vi "411x_Current _Chan Config Dialog.vi"(8 "error in (no error)":errorcluster, 10 "Item Ref out":T1=18446744073709551615 format="%.0x", 11 "Data Entry Limits:Maximum":dbl) -> (0 "error out":errorcluster, 1 "sense (out)":T2=1008 items=["Local"=1008, "Remote"=1009], 2 "Voltage Limit (out)":dbl, 3 "Initial Current Value (out)":dbl, 4 "Cancel (out)":bool, 5 "Number of Current Channels to Add? (out)":i16, 7 "Item Ref out":T1 format="%.0x")   [LabVIEW 2023, in "NI PXIe-411x PS Custom Device.lvlib"]
uses:
  NI PXIe-411x PS Custom Device.lvlib
  <instrlib>/niDCPower/nidcpower.llb/niDCPower Sense.ctl
  <vilib>/NI VeriStand/Custom Device API/Custom Device Item Ref.ctl
  411x_Global.vi
  <vilib>/NI VeriStand/Custom Device API/Get Item Property (Boolean).vi
  <vilib>/NI VeriStand/Custom Device API/Custom Device API.lvlib
panel:
  in  "Cancel":bool
  in  "OK Button":bool
  in  "Voltage Limit":dbl format="%.4f"
  in  "Initial Current Value":dbl
  in  "sense":T2=1008 caption="Sense" items=["Local"=1008, "Remote"=1009]
  in  "Number of Current Channels to Add?":i16
  # "Current Channels"
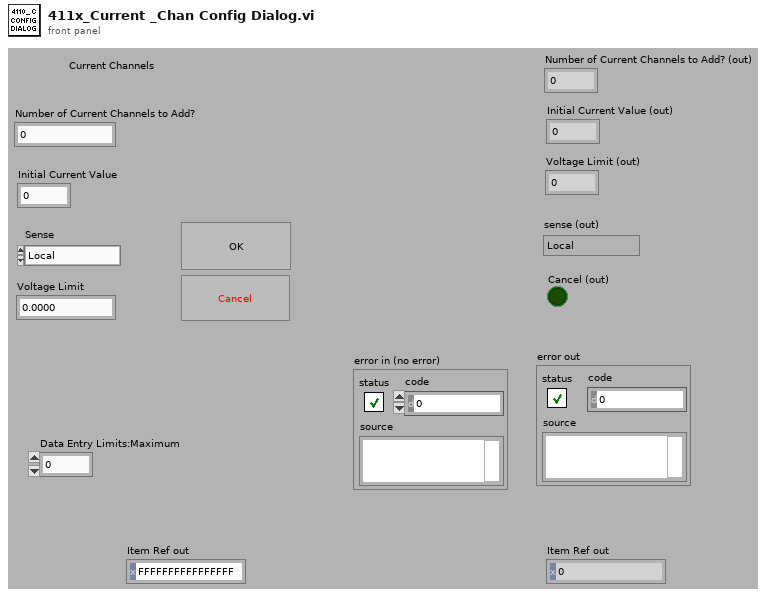
[diagram p1: front panel]
types:
  T1 = typedef "Custom Device API.lvlib/Custom Device Item Ref.ctl" = u64
  T2 = typedef "niDCPower Sense.ctl" = i32
  T3 = cluster{"V_min":dbl, "V_max":dbl, "I_min":dbl, "I_max":dbl}
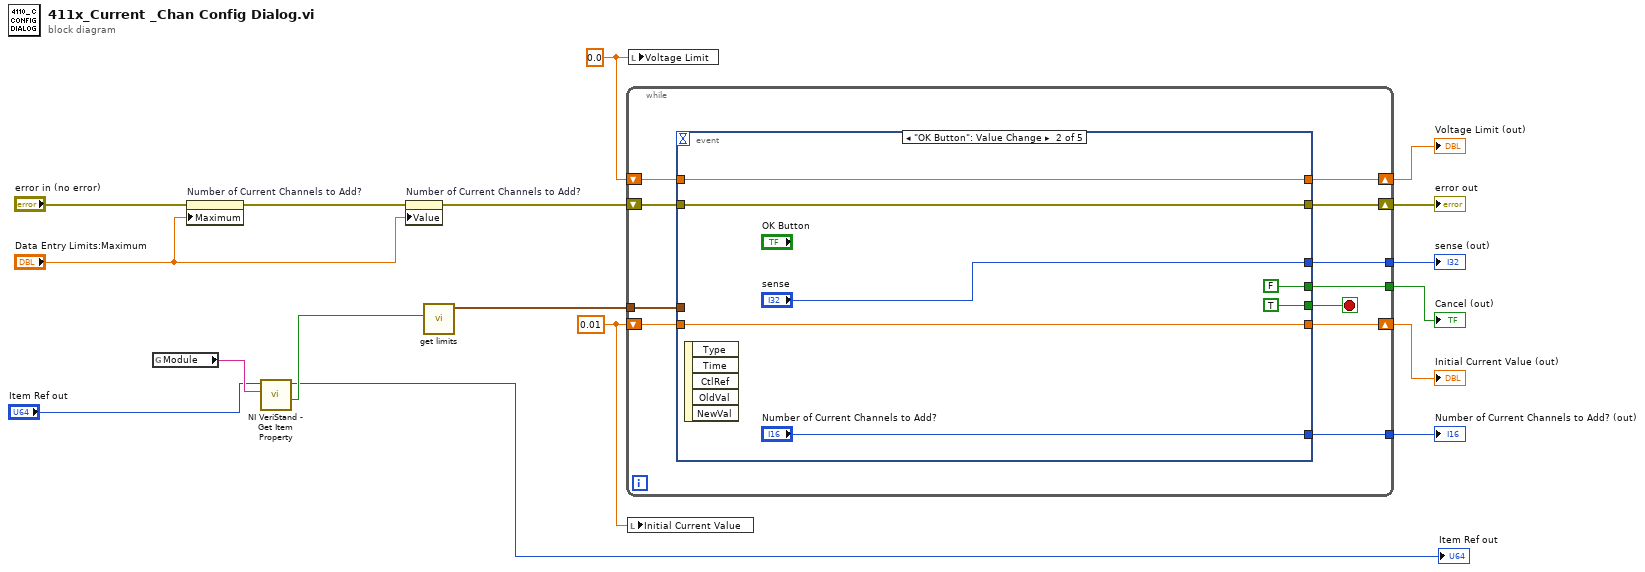
[diagram p0: block diagram]
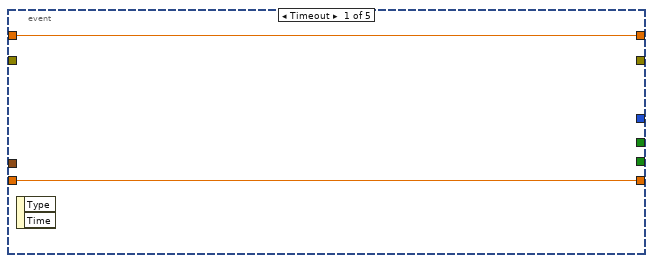
[diagram p2: hidden frame]
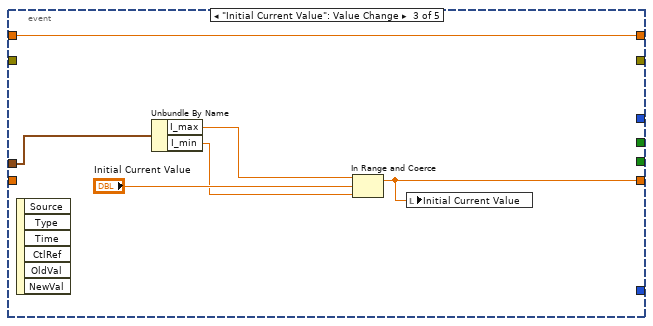
[diagram p3: hidden frame]
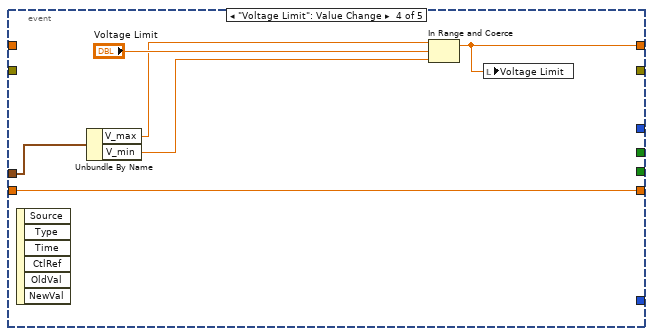
[diagram p4: hidden frame]
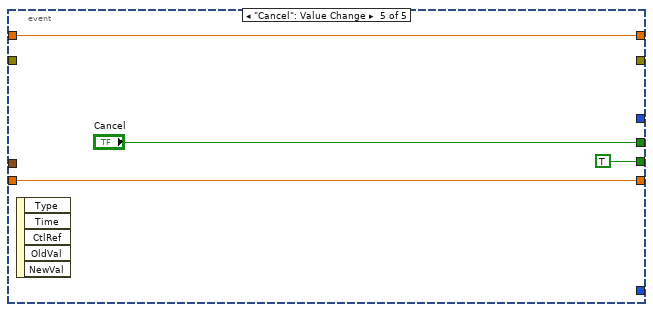
[diagram p5: hidden frame]
diagram:
  w7 = 0.0 ("Voltage Limit")
  w6 = 0.01 ("Initial Current Value")
  n1 = global read "411x_Global.vi" "Module"() -> (w5:string)
  n2 = property on="Number of Current Channels to Add?" class="DigNum (strict)"(error in="error in (no error)", "Maximum"="Data Entry Limits:Maximum") -> (error out=w17:errorcluster)  [unwired: 1 in, 1 out]
  n3 = call-poly <vilib>:"NI VeriStand - Get Item Property.vi"("Property Name"=w5, "Item Ref in"="Item Ref out") -> ("Value"=w3:bool, "Item Ref out"=→"Item Ref out":T1)  [unwired: 6 in, 2 out]
  n4 = property on="Number of Current Channels to Add?" class="DigNum (strict)"(error in=w17, "Value"="Data Entry Limits:Maximum") -> (error out=w15:errorcluster)  [unwired: 1 in, 1 out]
  n5 = call "get limits.vi"("4112?"=w3) -> ("output cluster"=w2:T3)  [unwired: 10 in]
  n6 = while {
    tunnel: [w25] -> w12
    tunnel: [w23] -> w10
    tunnel: [w22] -> w8
    shift-right: [w27] -> w14
    shift-left: w15 -> [w28]
    shift-right: [w24] -> w11
    shift-left: w6 -> [w20]
    shift-right: [w26] -> w13
    shift-left: w7 -> [w19]
    tunnel: w2 -> [w18]
    stop <- w21 stop-if-true
    n7 = event shown="[1] \"OK Button\": Value Change" {
      selector: _ -> [_ _ _ _ _]
      dyn-events: _ -> [_ _ _ _ _]
      timeout: _ -> [_ _ _ _ _]
      tunnel: [w29 w31 w42 w47 w50] -> w26
      tunnel: [_ "sense" _ _ _] -> w25
      tunnel: [w30 w32 w41 w49 w51] -> w24
      tunnel: w28 -> [_ w36 _ _ _]
      tunnel: [_ w36 _ _ _] -> w27
      tunnel: [_ FALSE ("Cancel") _ _ "Cancel"] -> w23
      tunnel: [_ "Number of Current Channels to Add?" _ _ _] -> w22
      tunnel: [_ TRUE ("Cancel") _ _ TRUE ("Cancel")] -> w21
      tunnel: w20 -> [w30 w32 _ w49 w51]
      tunnel: w19 -> [w29 w31 w42 _ w50]
      tunnel: w18 -> [_ _ w40 w46 _]
      event Timeout {
        n8 = event-data() -> ()  [unwired: 1 in, 2 out]
      }
      event "OK Button": Value Change {
        n9 = event-data() -> ()  [unwired: 1 in, 5 out]
      }
      event "Initial Current Value": Value Change {
        n10 = event-data() -> ()  [unwired: 1 in, 6 out]
        n11 = Unbundle By Name(w40) -> ("I_max"=w38:dbl, "I_min"=w39:dbl)
        n12 = In Range and Coerce(upper limit=w38, x="Initial Current Value", lower limit=w39) -> (coerced(x)=w41:dbl)  [unwired: 1 out]
        n13 = local write "Initial Current Value"(w41) -> ()
      }
      event "Voltage Limit": Value Change {
        n14 = event-data() -> ()  [unwired: 1 in, 6 out]
        n15 = Unbundle By Name(w46) -> ("V_max"=w45:dbl, "V_min"=w44:dbl)
        n16 = In Range and Coerce(upper limit=w45, x="Voltage Limit", lower limit=w44) -> (coerced(x)=w47:dbl)  [unwired: 1 out]
        n17 = local write "Voltage Limit"(w47) -> ()
      }
      event "Cancel": Value Change {
        n18 = event-data() -> ()  [unwired: 1 in, 5 out]
      }
    }
  }
  "error out" <- w14
  "Voltage Limit (out)" <- w13
  "sense (out)" <- w12
  "Initial Current Value (out)" <- w11
  "Cancel (out)" <- w10
  "Number of Current Channels to Add? (out)" <- w8
  n19 = local write "Initial Current Value"(w6) -> ()
  n20 = local write "Voltage Limit"(w7) -> ()
